vi "Compare Ports.vi"(9 "refresh listbox":T9[](array[typedef]), 10 "new port":T1={"hardware channel"=0, "direction"=enum."Rx", "labels"=[], "speed"=enum."HI (100 kb/s)"}, 11 "old port":T1={"hardware channel"=0, "direction"=enum."Rx", "labels"=[], "speed"=enum."HI (100 kb/s)"}) -> (1 "refresh listbox out":T9[](array[typedef]))   [LabVIEW 2020, in "AIM ARINC 429 System Explorer.lvlib" / "Implementation.lvlib"]
uses:
  Implementation.lvlib
  Types/Refresh Symbols.ctl
  Refresh Constants.vi
  <vilib>/NI/NI VeriStand Encoding and Decoding/Encoding.ctl
  <vilib>/NI/NI VeriStand Encoding and Decoding/Encoding and Decoding.lvlib
  Shared/Parameter Definition.ctl
  Shared/Direction.ctl
  Shared/VS Channel Definition for Parameter.ctl
  Shared/Transfer Type.ctl
  Shared/VS Channels Definition for Label.ctl
  Shared/VS Channels Definition for All Labels on Hardware Channel.ctl
  Types/Refresh Listbox.ctl
  Shared/Transfer Speed.ctl
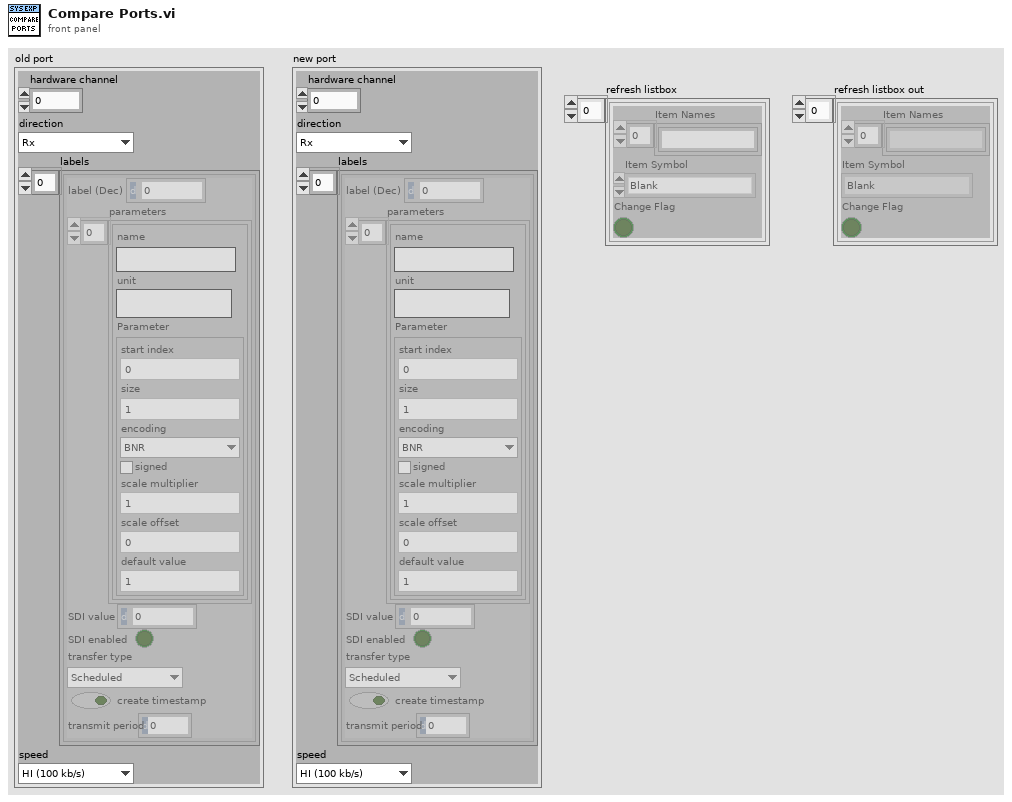
[diagram p1: front panel]
types:
  T1 = typedef "VS Channels Definition for All Labels on Hardware Channel.ctl" = cluster{"hardware channel":i32, "direction":T2, "labels":T3[], "speed":T8}
  T2 = typedef "Direction.ctl" = enum16{"Rx", "Tx"}
  T3 = typedef "VS Channels Definition for Label.ctl" = cluster{"label (Dec)":u32, "parameters":T4[], "SDI value":u8, "SDI enabled":bool, "transfer type":T7, "create timestamp":bool, "transmit period":u32}
  T4 = typedef "VS Channel Definition for Parameter.ctl" = cluster{"name":string, "unit":string, "Parameter":T5}
  T5 = typedef "Parameter Definition.ctl" = cluster{"start index":i32, "size":i32, "encoding":T6, "signed":bool, "scale multiplier":dbl, "scale offset":dbl, "default value":dbl}
  T6 = typedef "Encoding and Decoding.lvlib/Encoding.ctl" = enum16{"BNR", "BCD", "Discrete"}
  T7 = typedef "Transfer Type.ctl" = enum16{"Scheduled", "Acyclic", "Block", "Strobe"}
  T8 = typedef "Transfer Speed.ctl" = enum16{"LO (12.5 kb/s)", "HI (100 kb/s)"}
  T9 = typedef "AIM ARINC 429 System Explorer.lvlib/Implementation.lvlib/Refresh Listbox.ctl" = cluster{"Item Names":string[], "Item Symbol":T10, "Change Flag":bool}
  T10 = typedef "AIM ARINC 429 System Explorer.lvlib/Implementation.lvlib/Refresh Symbols.ctl" = enum16{"Blank", "Port", "Incoming", "Outgoing", "Label", "Word", "Parameter", "ARINC-429", "Config Files", "Channel Spec", "Item"}
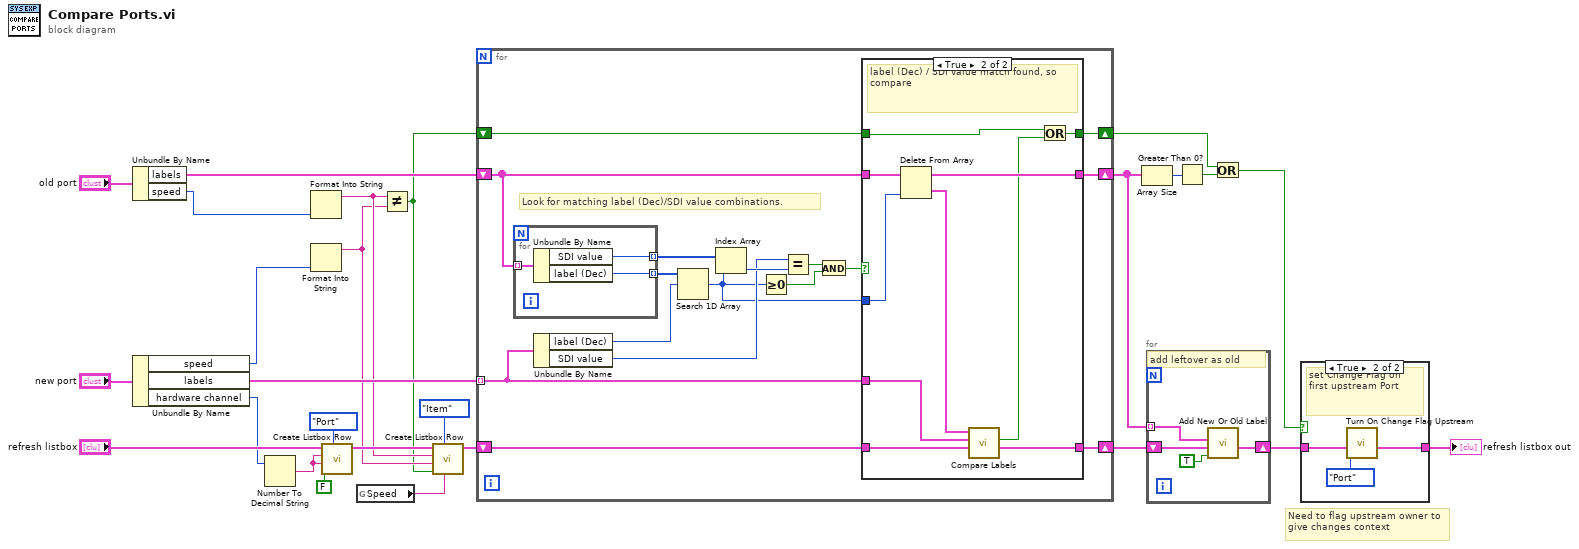
[diagram p0: block diagram]
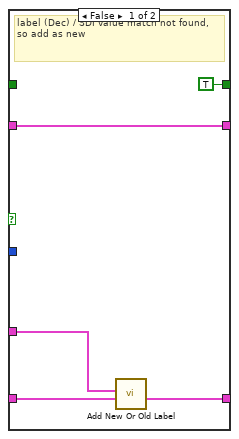
[diagram p3: hidden frame]
diagram:
  # "Need to flag upstream owner to give changes context"
  n1 = Unbundle By Name("old port") -> ("labels"=w20:T3[], "speed"=w7:T8)
  n2 = Unbundle By Name("new port") -> ("speed"=w6:T8, "labels"=w23:T3[], "hardware channel"=w22:i32)
  n3 = Number To Decimal String(number=w22) -> (decimal integer string=w19:string)  [unwired: 1 in]
  n4 = Format Into String(w7) -> (resulting string=w5:string)  [unwired: 3 in, 1 out]
  n5 = Format Into String(w6) -> (resulting string=w4:string)  [unwired: 3 in, 1 out]
  n6 = call "Create Listbox Row.vi"("refresh symbol (Blank)"=Refresh_Symbols."Port" ("Refresh Symbol (Blank)"), "change? (T)"=FALSE, "new item"=w19, "old item"=w19, "refresh listbox"="refresh listbox") -> ("refresh listbox out"=w8:T9[])  [unwired: 6 in]
  n7 = global read "Refresh Constants.vi" "Speed"() -> (w2:string)
  n8 = Not Equal?(x=w5, y=w4) -> (x != y?=w3:bool)
  n9 = call "Create Listbox Row.vi"("override name"=w2, "refresh symbol (Blank)"=Refresh_Symbols."Item", "change? (T)"=w3, "new item"=w4, "old item"=w5, "refresh listbox"=w8) -> ("refresh listbox out"=w9:T9[])  [unwired: 5 in]
  n10 = for {
    tunnel: w23 -> [w39] mode=indexing
    shift-right: [w41] -> w17
    shift-left: w9 -> [w42]
    shift-right: [w30] -> w14
    shift-left: w20 -> [w31]
    shift-right: [w27] -> w13
    shift-left: w3 -> [w28]
    # "Look for matching label (Dec)/SDI value combinations."
    n11 = for {
      tunnel: w31 -> [w60] mode=indexing
      tunnel: [w59] -> w40 mode=indexing
      tunnel: [w58] -> w37 mode=indexing
      n12 = Unbundle By Name(w60) -> ("SDI value"=w58:u8, "label (Dec)"=w59:u32)
    }
    n13 = Unbundle By Name(w39) -> ("label (Dec)"=w38:u32, "SDI value"=w35:u8)
    n14 = Search 1D Array(1D array=w40, element=w38) -> (index of element=w29:i32)  [unwired: 1 in]
    n15 = Index Array(array=w37, index=w29) -> (element=w36:u8)
    n16 = Greater Or Equal To 0?(x=w29) -> (x >= 0?=w33:bool)
    n17 = Equal?(x=w35, y=w36) -> (x = y?=w34:bool)
    n18 = And(x=w34, y=w33) -> (x .and. y?=w32:bool)
    n19 = case shown="True" w32 {
      tunnel: w42 -> [w44 w53]
      tunnel: [w45 w54] -> w41
      tunnel: w39 -> [w46 w52]
      tunnel: w31 -> [w47 w57]
      tunnel: [w47 w55] -> w30
      tunnel: w29 -> [_ w56]
      tunnel: w28 -> [_ w48]
      tunnel: [TRUE w50] -> w27
      frame False {
        # "label (Dec) / SDI value match not found, so add as new"
        n20 = call "Add New Or Old Label.vi"("refresh listbox"=w44, "label"=w46) -> ("refresh listbox out"=w45:T9[])  [unwired: 9 in]
      }
      frame True {
        # "label (Dec) / SDI value match found, so compare"
        n21 = Delete From Array(array=w57, index=w56) -> (deleted portion=w51:T3, array with subset deleted=w55:T3[])  [unwired: 1 in]
        n22 = call "Compare Labels.vi"("refresh listbox"=w53, "new label"=w52, "old label"=w51) -> ("refresh listbox out"=w54:T9[], "any changes?"=w49:bool)  [unwired: 7 in]
        n23 = Or(x=w48, y=w49) -> (x .or. y?=w50:bool)
      }
    }
  }
  n24 = Array Size(array=w14) -> (size(s)=w15:i32)
  n25 = for {
    shift-right: [w63] -> w12
    shift-left: w17 -> [w64]
    tunnel: w14 -> [w62] mode=indexing
    # "add leftover as old"
    n26 = call "Add New Or Old Label.vi"("old label?"=TRUE, "refresh listbox"=w64, "label"=w62) -> ("refresh listbox out"=w63:T9[])  [unwired: 8 in]
  }
  n27 = Greater Than 0?(x=w15) -> (x > 0?=w16:bool)
  n28 = Or(x=w13, y=w16) -> (x .or. y?=w11:bool)
  n29 = case shown="True" w11 {
    tunnel: w12 -> [w65 w68]
    tunnel: [w65 w67] -> w10
    frame False {
    }
    frame True {
      # "set Change Flag on first upstream Port"
      n30 = call "Turn On Change Flag Upstream.vi"("symbol to change"=Refresh_Symbols."Port", "refresh listbox"=w68) -> ("refresh listbox out"=w67:T9[])  [unwired: 9 in]
    }
  }
  "refresh listbox out" <- w10
